vi "Calculate Drive Speeds.vi"(0 "Left Speed In":dbl, 1 "Right Speed In":dbl) -> (4 "Front Left Speed":dbl, 5 "Front Right Speed":dbl, 6 "Rear Left Speed":dbl, 7 "Rear Right Speed":dbl)   [LabVIEW 2011]
uses:
  Globals/Max Robot Speed.vi
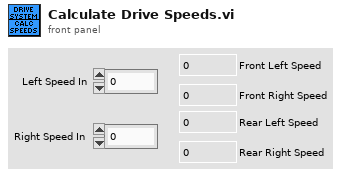
[diagram p1: front panel]
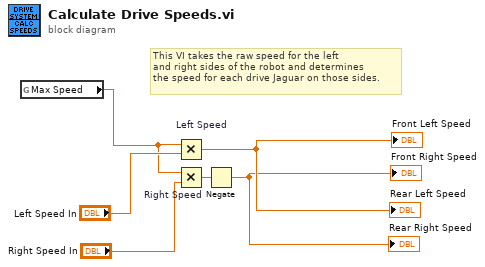
[diagram p0: block diagram]
diagram:
  # "This VI takes the raw speed for the left\nand right sides of the robot and determines\nthe speed for each drive Jaguar on those sides."
  n1 = global read "Max Robot Speed.vi" "Max Speed"() -> (w1:dbl)
  n2 = Multiply "Left Speed"(x=w1, y="Left Speed In") -> (x*y=→"Rear Left Speed" →"Front Left Speed":dbl)
  n3 = Multiply "Right Speed"(x=w1, y="Right Speed In") -> (x*y=w4:dbl)
  n4 = Negate(x=w4) -> (-x=→"Front Right Speed" →"Rear Right Speed":dbl)
